vi "Read (Multiple Points).vi"(8 "error in (no error)":errorcluster, 9 "Timeout (10000 ms)":i32=10000 format="%#.6g", 10 "Sample Count (1)":i32=1, 11 "VISA resource name":refnum<visa-resource-name>) -> (0 "error out":errorcluster, 2 "Measurements":dbl[](array[numeric]), 3 "VISA resource name out":refnum<visa-resource-name>)   [LabVIEW 2011, in "Template - DMM.lvlib"]
doc: "Reads and returns multiple measurements from the instrument. Use this VI when you want to take multiple measurements using an immediate trigger. Use the low-level VIs for other triggering options."
uses:
  <instrlib>/_Template - DMM/Template - DMM.lvlib
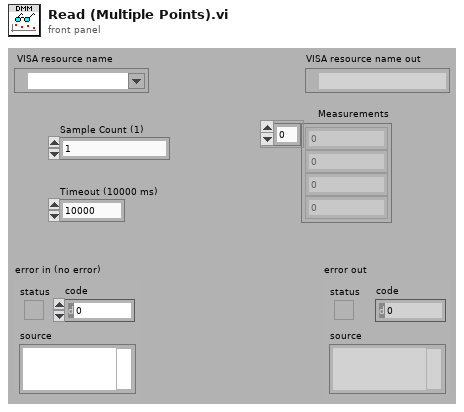
[diagram p1: front panel]
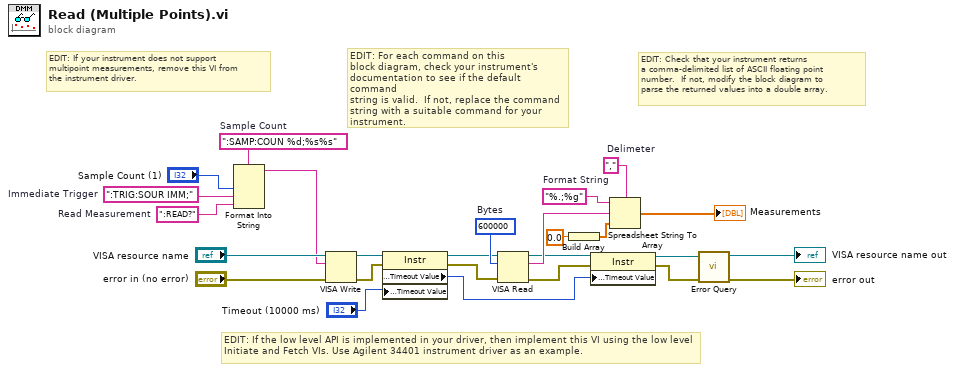
[diagram p0: block diagram]
diagram:
  w1 = ":TRIG:SOUR IMM;"  # Immediate Trigger
  w5 = ":SAMP:COUN %d;%s%s"  # Sample Count
  w19 = ","  # Delimeter
  w20 = "%.;%g"  # Format String
  w2 = ":READ?"  # Read Measurement
  w26 = u32 600000  # Bytes
  # "EDIT: If the low level API is implemented in your driver, then implement this VI using the low level Initiate and Fetch VIs. Use Agilent 34401 instrument driver as an example."
  # "EDIT: If your instrument does not support\nmultipoint measurements, remove this VI from\nthe instrument driver."
  # "EDIT: Check that your instrument returns\na comma-delimited list of ASCII floating point\nnumber.  If not, modify the block diagram to\nparse the returned values into a double array."
  # "EDIT: For each command on this\nblock diagram, check your instrument's\ndocumentation to see if the default command\nstring is valid.  If not, replace the command\nstring with a suitable command for your\ninstrument."
  n1 = Format Into String(format string=w5, "Sample Count (1)", w1, w2) -> (resulting string=w3:string)  [unwired: 2 in, 1 out]
  n2 = VISA Write(VISA resource name="VISA resource name", write buffer=w3, error in (no error)="error in (no error)") -> (VISA resource name out=w15:refnum<visa-resource-name>, error out=w14:errorcluster)  [unwired: 1 out]
  n3 = property class="Instr"(reference=w15, error in=w14, "General Settings:Timeout Value"="Timeout (10000 ms)") -> (reference out=w13:refnum<visa-resource-name>, error out=w12:errorcluster, "General Settings:Timeout Value"=w6:u32)
  n4 = VISA Read(VISA resource name=w13, byte count=w26, error in (no error)=w12) -> (VISA resource name out=w10:refnum<visa-resource-name>, read buffer=w21:string, error out=w8:errorcluster)  [unwired: 1 out]
  n5 = Build Array(0.0) -> (w17:dbl[])
  n6 = property class="Instr"(reference=w10, error in=w8, "General Settings:Timeout Value"=w6) -> (reference out=w9:refnum<visa-resource-name>, error out=w7:errorcluster)
  n7 = Spreadsheet String To Array(delimiter (Tab)=w19, format string=w20, spreadsheet string=w21, array type (2D Dbl)=w17) -> (array=→"Measurements":dbl[])
  n8 = call <instrlib>:"Error Query.vi"("error in (no error)"=w7, "VISA resource name"=w9) -> ("error out"=→"error out":errorcluster, "VISA resource name out"=→"VISA resource name out":refnum<visa-resource-name>)  [unwired: 6 in, 2 out]
